vi "GetFileTree.vi"(9 "Tree":refnum<vi>, 10 "Open?":bool, 11 "Base Path":path) -> ()   [LabVIEW 2020]
panel:
  in  "Tree":string(tree)
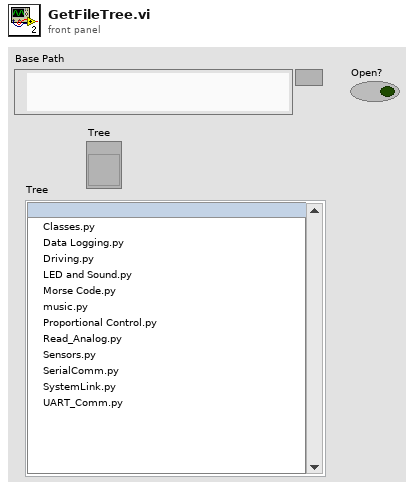
[diagram p1: front panel]
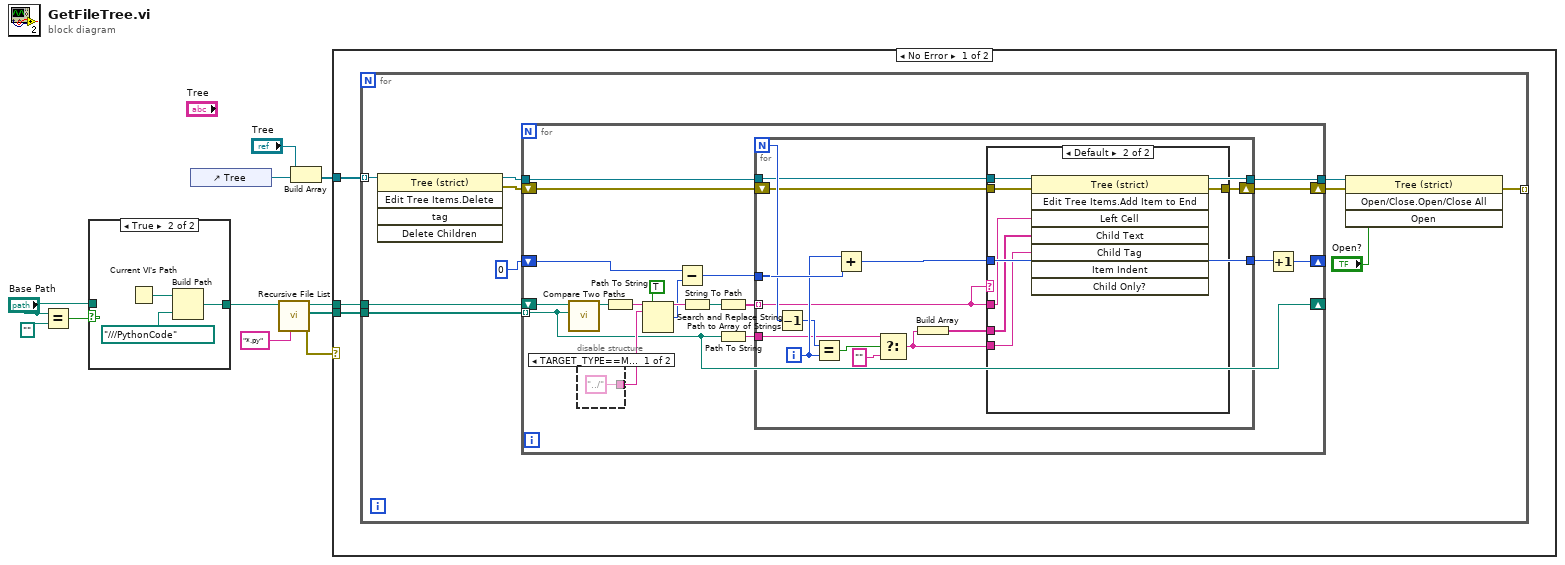
[diagram p0: block diagram]
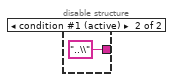
[diagram p3: hidden frame]
diagram:
  n1 = Equal?(x="Base Path", y=path "") -> (x = y?=w7:bool)
  n2 = case shown="True" w7 {
    tunnel: [w12 w13] -> w3
    tunnel: "Base Path" -> [w12 _]
    frame False {
    }
    frame True {
      n3 = Current VI's Path() -> (path=w15:path)
      n4 = Build Path(base path=w15, name or relative path=path "../../../PythonCode") -> (appended path=w13:path)
    }
  }
  n5 = control-ref of="Tree"() -> (w4:refnum<vi>)
  n6 = call <vilib>:"Recursive File List.vi"("pattern"="*.py", "Folder Path"=w3) -> ("error out"=w9:errorcluster, "All Files in Dir"=w11:path[], "dup Folder Path"=w2:path)  [unwired: 5 in, 2 out]
  n7 = Build Array("Tree", w4) -> (w1:refnum<vi>[])
  n8 = case shown="No Error" w9 {
    tunnel: w1 -> [w18 _]
    tunnel: w11 -> [w17 _]
    tunnel: w2 -> [w16 _]
    frame No Error {
      n9 = for {
        tunnel: w18 -> [w28] mode=indexing
        tunnel: w17 -> [w26]
        tunnel: w16 -> [w25]
        tunnel: [w19] -> _ mode=indexing
        n10 = invoke on="Invoke Node" class="Tree (strict)" method="Edit Tree Items.Delete"(reference=w28) -> (reference out=w24:refnum<vi>, error out=w21:errorcluster)  [unwired: 4 in, 3 out]
        n11 = for {
          tunnel: w26 -> [w34] mode=indexing
          shift-right: [w34] -> _
          shift-left: w25 -> [w47]
          shift-right: [w35] -> _
          shift-left: 0 -> [w37]
          tunnel: w24 -> [w32]
          tunnel: [w31] -> w22
          shift-right: [w29] -> w20
          shift-left: w21 -> [w30]
          n12 = call <vilib>:"Compare Two Paths.vi"("Path 2"=w34, "Path 1"=w47) -> ("Relative Path from 1 to 2"=w39:path)  [unwired: 6 in, 3 out]
          n13 = disable-structure shown="TARGET_TYPE==Mac" {
            disable-tunnel: ["../" ("search string") "..\\" ("search string")] -> w45
            frame condition #0 {
            }
            frame condition #1 (active) {
            }
          }
          n14 = Path To String(path=w39) -> (string=w46:string)
          n15 = Search and Replace String(replace all?=TRUE ("replace all? (F)"), input string=w46, search string=w45) -> (result string=w43:string, number of replacements=w40:i32)  [unwired: 5 in, 2 out]
          n16 = Subtract(x=w37, y=w40) -> (x-y=w38:i32)
          n17 = String To Path(string=w43) -> (path=w42:path)
          n18 = Path to Array of Strings(0:w42) -> (2:w41:string[])  [unwired: 1 out]
          n19 = Path To String(path=w34) -> (string=w33:string)
          n20 = for {
            N -> [w60]
            tunnel: w41 -> [w52] mode=indexing
            tunnel: w38 -> [w63]
            tunnel: [w62] -> w36
            tunnel: w33 -> [w54]
            tunnel: w32 -> [w51]
            tunnel: [w51] -> w31
            shift-right: [w53] -> w29
            shift-left: w30 -> [w50]
            i -> [w61]
            n21 = Decrement(x=w60) -> (x-1=w59:i32)
            n22 = Equal?(x=w59, y=w61) -> (x = y?=w58:bool)
            n23 = Add(x=w61, y=w63) -> (x+y=w62:i32)
            n24 = Select(t=w54, s=w58, f="") -> (s? t:f=w56:string)
            n25 = Build Array(w56) -> (w55:string[])
            n26 = case shown="Default" w52 {
              tunnel: w52 -> [_ w70]
              tunnel: w62 -> [_ w69]
              tunnel: w56 -> [_ w68]
              tunnel: w55 -> [_ w67]
              tunnel: [_ w66] -> w53
              tunnel: w51 -> [_ w65]
              tunnel: w50 -> [_ w64]
              frame ".DS_Store" {
              }
              frame Default {
                n27 = invoke on="Invoke Node" class="Tree (strict)" method="Edit Tree Items.Add Item to End"(reference=w65, error in=w64, "Left Cell"=w70, "Child Text"=w67, "Child Tag"=w68, "Item Indent"=w69) -> (error out=w66:errorcluster)  [unwired: 2 in, 7 out]
              }
            }
          }
          n28 = Increment(x=w36) -> (x+1=w35:i32)
        }
        n29 = invoke on="Invoke Node" class="Tree (strict)" method="Open/Close.Open/Close All"(reference=w22, error in=w20, "Open"="Open?") -> (error out=w19:errorcluster)  [unwired: 1 in, 3 out]
      }
    }
    frame Error {
    }
  }
